vi "Embedded Project v3.vi"() -> ()   [LabVIEW 2015]
uses:
  <vilib>/Instr/_visa.llb/Select Event Type.ctl
  <vilib>/Instr/_visa.llb/VISA Configure Serial Port (Instr).vi
panel:
  in  "Tab Control":enum32{"Main", "Settings"}(tab)
  out "Node 3 Status":bool
  out "Node 2 Status":bool
  out "Bridge Stress":dbl[][](graph)
  out "Node 1 Status":bool
  out "Z Axis":dbl[][](graph)
  out "Y Axis":dbl[][](graph)
  out "X Axis":dbl[][](graph)
  out "Node 1 Water Level":u8(knob) scale=0.0..3.0
  out "Node 2 Water Level":u8(knob) scale=0.0..3.0
  out "Node 3 Water Level":u8(knob) scale=0.0..3.0
  out "Earthquake\nWarning":bool
  out "Tsunami \nWarning":bool
  out "Structure\nWarning":bool
  out "Serial Monitor":string
  out "System Time":string
  in  "COM Port":refnum<visa-resource-name>="COM1"
  in  "Terminate":bool
  out "Data Sorting":T1(array[cluster])
  out "New Serial Data":string
  # "Water Level Monitoring"
  # "Sensor Node Status"
  # "Earthquake Monitoring"
  # "Bridge Health Monitoring"
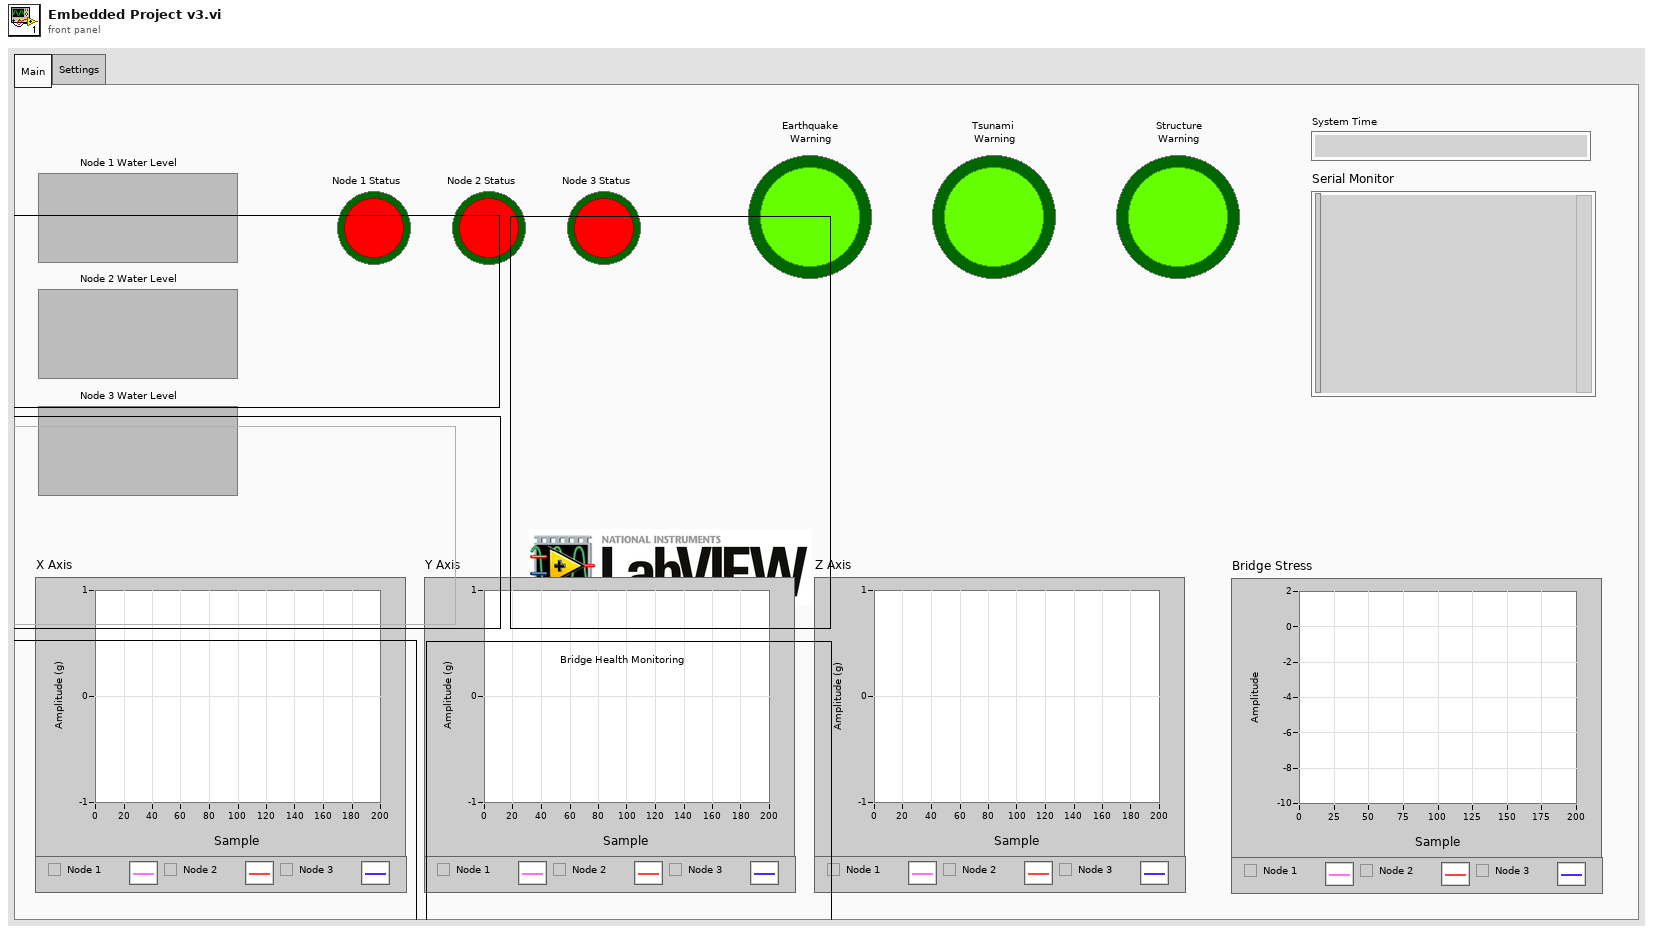
[diagram p1: front panel]
types:
  T1 = cluster{"Node Address":u16, "Water Level":i16, "Load Cell":i16, "Z Axis":i16, "Y Axis":i16, "X Axis":i16, "Status":u8}[]
  T2 = cluster{"Node Address":u16, "Water Level":i16, "Load Cell":i16, "X Axis":i16, "Y Axis":i16, "Z Axis":i16, "Status":u8}[]
  T3 = typedef "Select Event Type.ctl" = u32
  T4 = cluster{"baud rate (9600)":u32, "data bits (8)":u16, "parity (0:none)":enum16{"None", "Odd", "Even", "Mark", "Space"}, "stop bits (10: 1 bit)":u16, "flow control (0:none)":u16}
  T5 = cluster{"Node Address":u16, "Water Level":i16, "Load Cell":i16, "X Axis":i16, "Y Axis":i16, "Z Axis":i16, "Status":u8}
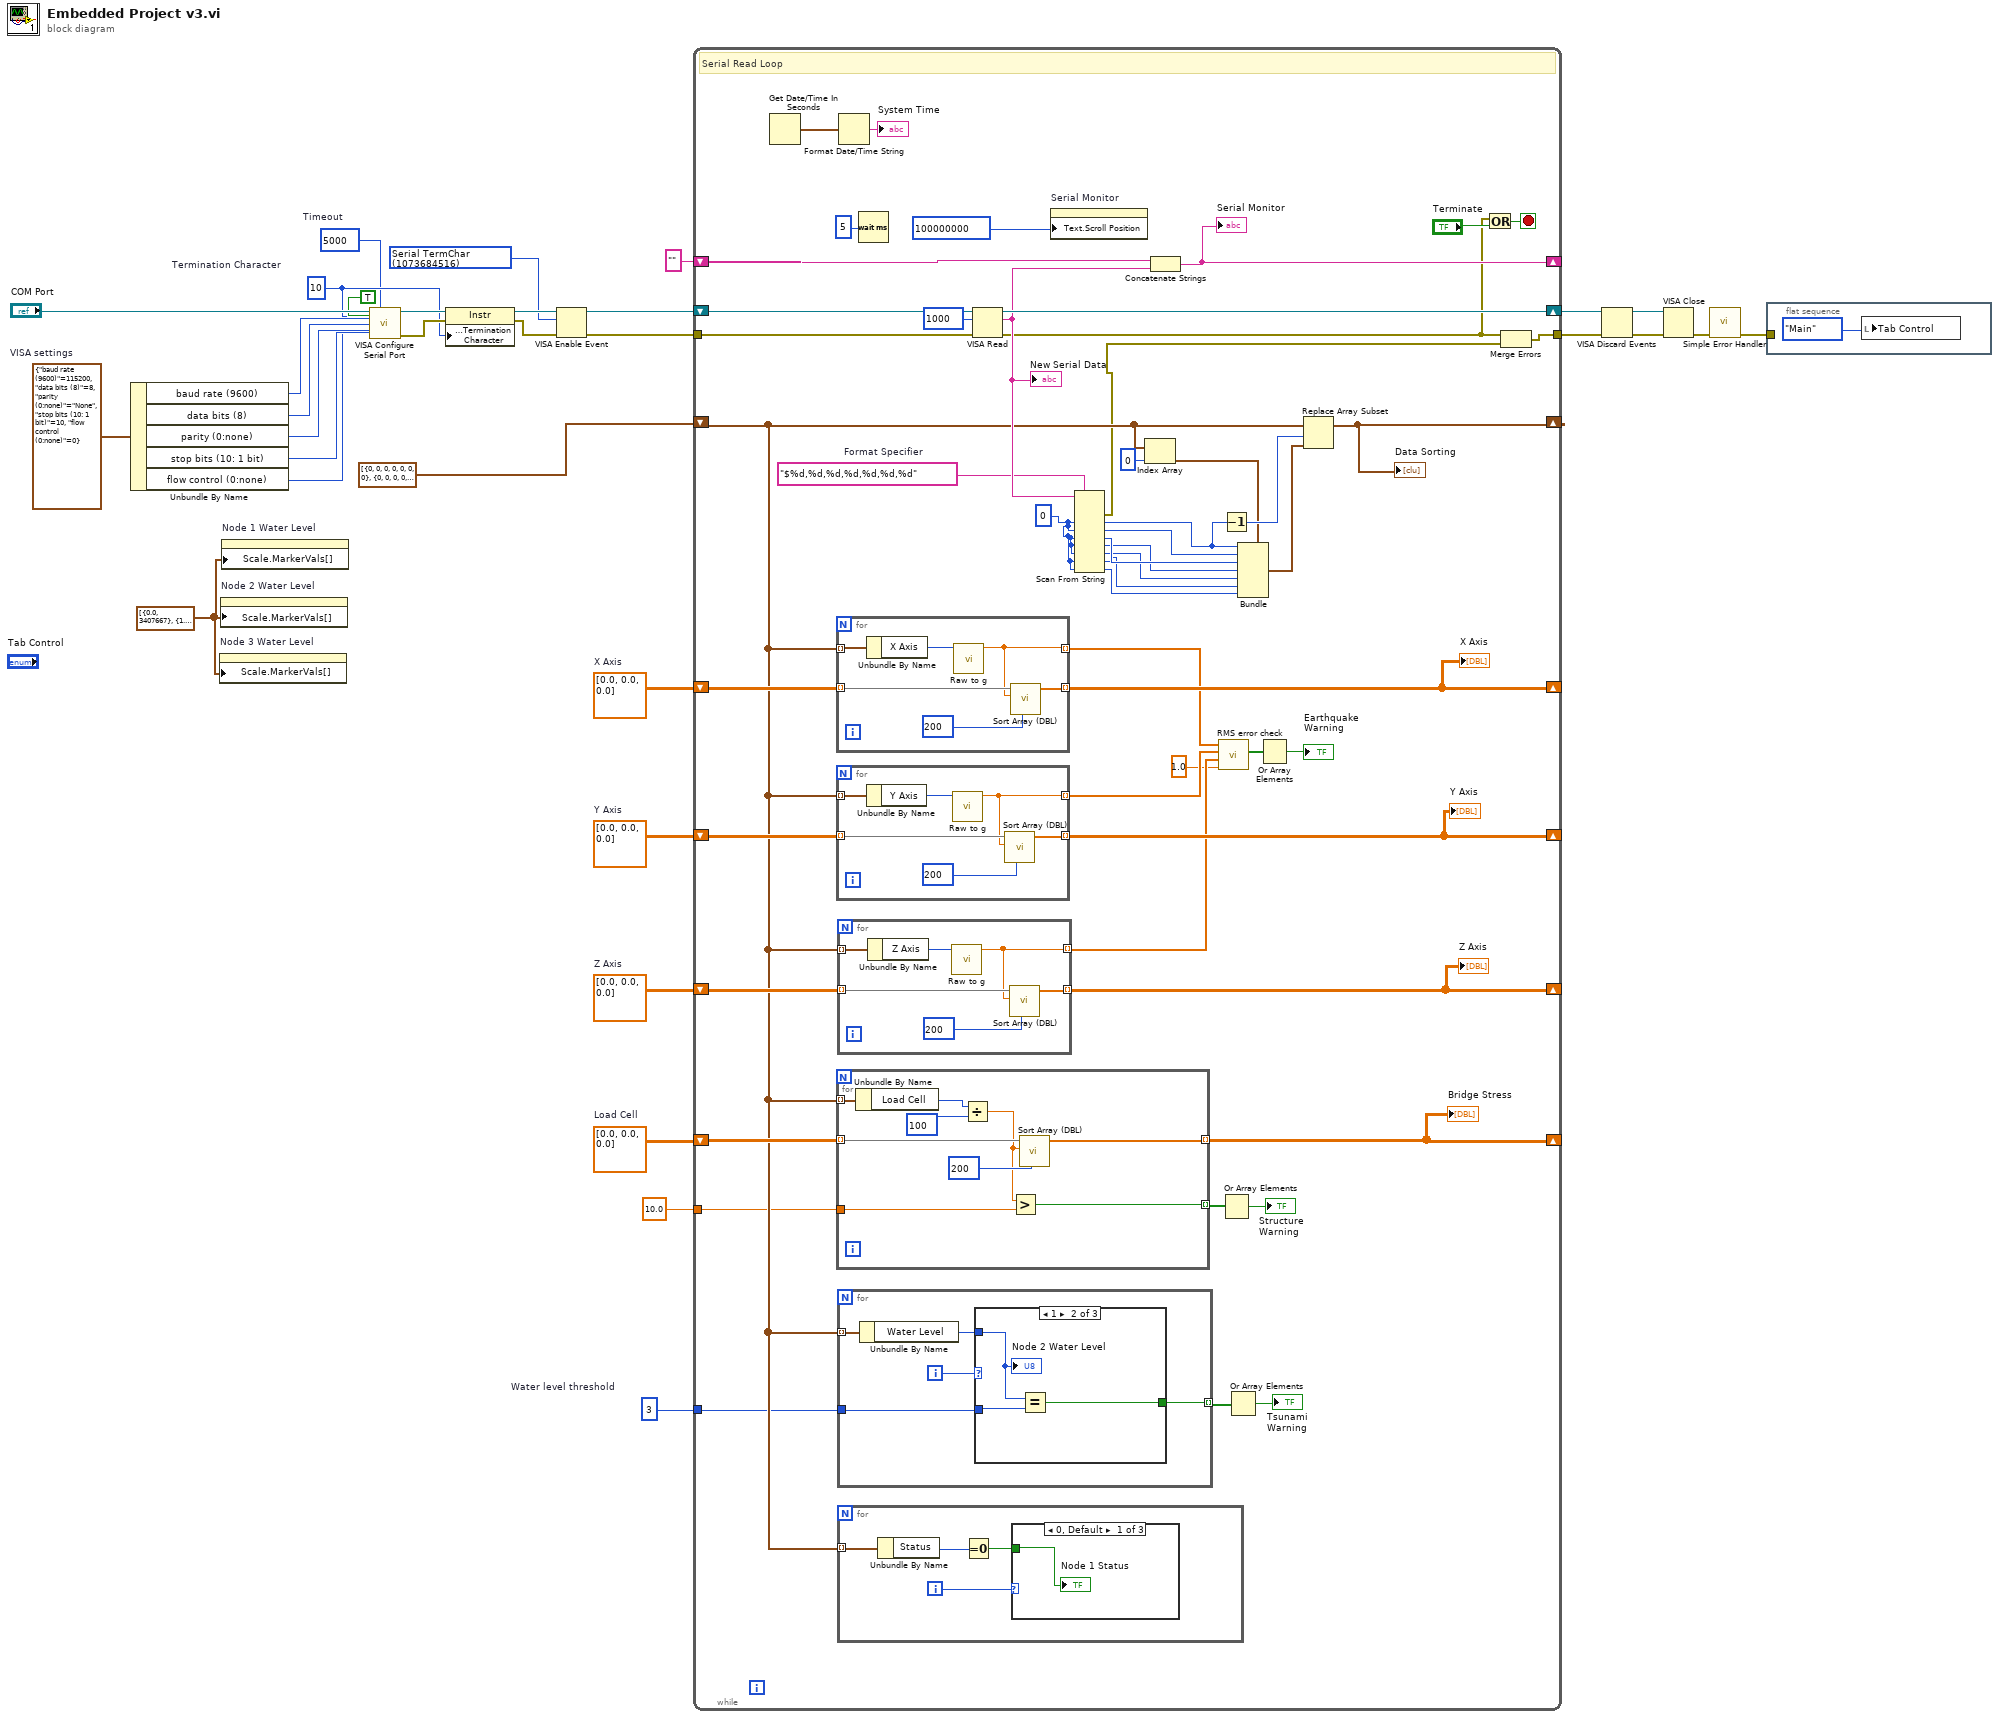
[diagram p0: block diagram]
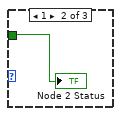
[diagram p2: hidden frame]
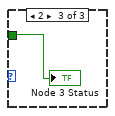
[diagram p3: hidden frame]
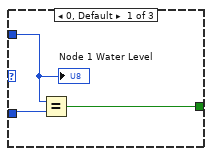
[diagram p4: hidden frame]
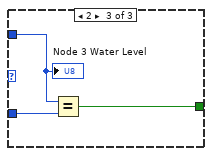
[diagram p5: hidden frame]
diagram:
  w2 = i16 3  # Water level threshold
  w3 = u32 5000  # Timeout
  w7 = cluster{dbl, u32}[] [{0.0, 3407667}, {1.0, 16777011}, {2.0, 16750899}, {3.0, 13369344}] ("Scale.Marker Values[]")
  w8 = dbl[][] [[0.0], [0.0], [0.0]]  # Load Cell
  w10 = dbl[][] [[0.0], [0.0], [0.0]]  # Z Axis
  w11 = dbl[][] [[0.0], [0.0], [0.0]]  # Y Axis
  w12 = dbl[][] [[0.0], [0.0], [0.0]]  # X Axis
  w18 = T3 1073684516 items=["Service Request"=1073684491, "Trigger"=3221168138, "Clear"=1073684493, "VXI Signal"=1073684512, "VXI/VME Interrupt"=3221168161, "VXI/VME Sysfail"=1073684509, "VXI/VME Sysreset"=1073684510, "GPIB CIC"=1073684498, "GPIB Talk"=1073684499, "GPIB Listen"=1073684500, "PXI Interrupt"=1073684514, "Serial Break"=1073684515, "Serial TermChar"=1073684516, "Serial CTS"=1073684521, "Serial DSR"=1073684522, "Serial DCD"=1073684524, "Serial RI"=1073684526, "Serial Character"=1073684533, "USB Interrupt"=1073684535, "All Enabled"=1073709055] ("Event Type")
  w28 = T4 {"baud rate (9600)"=115200, "data bits (8)"=8, "parity (0:none)"=enum."None", "stop bits (10: 1 bit)"=10, "flow control (0:none)"=0}  # VISA settings
  w21 = u8 10  # Termination Character
  n1 = Unbundle By Name(w28) -> ("baud rate (9600)"=w27:u32, "data bits (8)"=w26:u16, "parity (0:none)"=w25:enum16{"None", "Odd", "Even", "Mark", "Space"}, "stop bits (10: 1 bit)"=w24:u16, "flow control (0:none)"=w23:u16)
  n2 = property on="Node 3 Water Level" class="Knob (strict)"("Scale.MarkerVals[]"=w7) -> ()  [unwired: 2 in, 2 out]
  n3 = property on="Node 2 Water Level" class="Knob (strict)"("Scale.MarkerVals[]"=w7) -> ()  [unwired: 2 in, 2 out]
  n4 = property on="Node 1 Water Level" class="Knob (strict)"("Scale.MarkerVals[]"=w7) -> ()  [unwired: 2 in, 2 out]
  n5 = call-poly "VISA Configure Serial Port"("VISA resource name"="COM Port", "timeout (10sec)"=w3, "termination char\n(0xA = '\\n' = LF)"=w21, "Enable Termination\nChar (T)"=TRUE ("End Read on Termination Character?"), "baud rate (9600)"=w27, "data bits (8)"=w26, "parity (0:none)"=w25, "stop bits (10: 1 bit)"=w24, "flow control (0:none)"=w23) -> ("VISA resource name out"=w31:refnum<visa-resource-name>, "error out"=w22:errorcluster)  [unwired: 1 in, 4 out]
  n6 = property class="Instr"(reference=w31, error in=w22, "Message Based Settings:Termination Character"=w21) -> (reference out=w19:refnum<visa-resource-name>, error out=w20:errorcluster)
  n7 = VISA Enable Event(8:w20, 10:w18, 11:w19) -> (0:w5:errorcluster, 3:w6:refnum<visa-resource-name>)  [unwired: 1 in]
  n8 = while {
    shift-right: [w83] -> w16
    shift-left: w6 -> [w65]
    tunnel: [w50] -> w13
    shift-right: [w78] -> _
    shift-left: "" -> [w79]
    shift-right: [w76] -> _
    shift-left: T2 [{"Node Address"=0, "Water Level"=0, "Load Cell"=0, "X Axis"=0, "Y Axis"=0, "Z Axis"=0, "Status"=0}, {"Node Address"=0, "Water Level"=0, "Load Cell"=0, "X Axis"=0, "Y Axis"=0, "Z Axis"=0, "Status"=0}, {"Node Address"=0, "Water Level"=0, "Load Cell"=0, "X Axis"=0, "Y Axis"=0, "Z Axis"=0, "Status"=0}] ("Array") -> [w53]
    shift-right: [w46] -> _
    shift-left: w12 -> [w75]
    shift-right: [w47] -> _
    shift-left: w11 -> [w74]
    shift-right: [w45] -> _
    shift-left: w10 -> [w73]
    shift-right: [w70] -> _
    shift-left: w8 -> [w71]
    tunnel: w5 -> [w64]
    tunnel: w2 -> [w44]
    tunnel: 10.0 ("y") -> [w41]
    stop <- w81 stop-if-true
    w60 = i16 0 ("default value 1")
    w67 = "$%d,%d,%d,%d,%d,%d,%d"  # Format Specifier
    # "Serial Read Loop"
    n9 = Get Date/Time In Seconds() -> (seconds since 1Jan1904=w69:timestamp)
    n10 = for {
      tunnel: w53 -> [w131] mode=indexing
      tunnel: w75 -> [w129] mode=indexing
      tunnel: [w128] -> w46 mode=indexing
      tunnel: [w126] -> w38 mode=indexing
      n11 = Unbundle By Name(w131) -> ("X Axis"=w130:i16)
      n12 = call "Raw to g.vi"("Input"=w130) -> ("Output"=w126:dbl)  [unwired: 10 in]
      n13 = call "Sort Array (DBL).vi"("Max Size"=200, "New Element"=w126, "Array In"=w129) -> ("Array Out"=w128:dbl[])  [unwired: 8 in]
    }
    "X Axis" <- w46
    n14 = for {
      tunnel: w74 -> [w123] mode=indexing
      tunnel: w53 -> [w125] mode=indexing
      tunnel: [w122] -> w47 mode=indexing
      tunnel: [w120] -> w37 mode=indexing
      n15 = Unbundle By Name(w125) -> ("Y Axis"=w124:i16)
      n16 = call "Raw to g.vi"("Input"=w124) -> ("Output"=w120:dbl)  [unwired: 10 in]
      n17 = call "Sort Array (DBL).vi"("Max Size"=200, "New Element"=w120, "Array In"=w123) -> ("Array Out"=w122:dbl[])  [unwired: 8 in]
    }
    "Y Axis" <- w47
    n18 = for {
      tunnel: [w112] -> w70 mode=indexing
      tunnel: w71 -> [w111] mode=indexing
      tunnel: w53 -> [w113] mode=indexing
      tunnel: w41 -> [w106]
      tunnel: [w105] -> w40 mode=indexing
      n19 = Unbundle By Name(w113) -> ("Load Cell"=w109:i16)
      n20 = Divide(x=w109, y=i16 100) -> (x/y=w107:dbl)
      n21 = Greater?(x=w107, y=w106) -> (0:w105:bool)
      n22 = call "Sort Array (DBL).vi"("Max Size"=200, "New Element"=w107, "Array In"=w111) -> ("Array Out"=w112:dbl[])  [unwired: 8 in]
    }
    "Bridge Stress" <- w70
    n23 = for {
      tunnel: w73 -> [w117] mode=indexing
      tunnel: w53 -> [w119] mode=indexing
      tunnel: [w116] -> w45 mode=indexing
      tunnel: [w114] -> w36 mode=indexing
      n24 = Unbundle By Name(w119) -> ("Z Axis"=w118:i16)
      n25 = call "Raw to g.vi"("Input"=w118) -> ("Output"=w114:dbl)  [unwired: 10 in]
      n26 = call "Sort Array (DBL).vi"("Max Size"=200, "New Element"=w114, "Array In"=w117) -> ("Array Out"=w116:dbl[])  [unwired: 8 in]
    }
    "Z Axis" <- w45
    n27 = for {
      tunnel: w53 -> [w95] mode=indexing
      tunnel: w44 -> [w92]
      tunnel: [w91] -> w43 mode=indexing
      i -> [w94]
      n28 = Unbundle By Name(w95) -> ("Water Level"=w93:i16)
      n29 = case shown="1" w94 {
        tunnel: w93 -> [w98 w101 w104]
        tunnel: w92 -> [w96 w99 w103]
        tunnel: [w97 w100 w102] -> w91
        frame 0, Default {
          n30 = Equal?(x=w98, y=w96) -> (x = y?=w97:bool)
          "Node 1 Water Level" <- w98
        }
        frame 1 {
          n31 = Equal?(x=w101, y=w99) -> (x = y?=w100:bool)
          "Node 2 Water Level" <- w101
        }
        frame 2 {
          n32 = Equal?(x=w104, y=w103) -> (x = y?=w102:bool)
          "Node 3 Water Level" <- w104
        }
      }
    }
    n33 = for {
      tunnel: w53 -> [w87] mode=indexing
      i -> [w86]
      n34 = Unbundle By Name(w87) -> ("Status"=w85:u8)
      n35 = Equal To 0?(x=w85) -> (x = 0?=w84:bool)
      n36 = case shown="0, Default" w86 {
        tunnel: w84 -> [w88 w89 w90]
        frame 0, Default {
          "Node 1 Status" <- w88
        }
        frame 1 {
          "Node 2 Status" <- w89
        }
        frame 2 {
          "Node 3 Status" <- w90
        }
      }
    }
    n37 = Format Date/Time String(seconds (now)=w69) -> (date/time string=→"System Time":string)  [unwired: 2 in]
    n38 = Wait (ms)(milliseconds to wait=u32 5) -> ()  [unwired: 1 out]
    n39 = VISA Read(VISA resource name=w65, byte count=u32 1000, error in (no error)=w64) -> (VISA resource name out=w83:refnum<visa-resource-name>, read buffer=w77:string, error out=w49:errorcluster)  [unwired: 1 out]
    "New Serial Data" <- w77
    n40 = property on="Serial Monitor" class="Str"("Text.Scroll Position"=u32 100000000) -> ()  [unwired: 2 in, 2 out]
    n41 = Scan From String(format string=w67, input string=w77, default 1=w60, default 2=w60, default 3=w60, default 4=w60, default 5=w60, default 6=w60, default 7=w60) -> (error out=w48:errorcluster, output 1=w66:i16, output 2=w59:i16, output 3=w58:i16, output 4=w57:i16, output 5=w56:i16, output 6=w55:i16, output 7=w54:i16)  [unwired: 2 in, 2 out]
    n42 = Index Array(array=w53, index=0) -> (element=w51:T5)
    n43 = Concatenate Strings(w79, w77) -> (w78:string)
    "Serial Monitor" <- w78
    n44 = call "RMS error check.vi"("Threshold"=1.0, "Z Axis"=w36, "Y Axis"=w37, "X Axis"=w38) -> ("Error?"=w34:bool[])  [unwired: 6 in, 1 out]
    n45 = Decrement(x=w66) -> (x-1=w62:i16)
    n46 = Or Array Elements(Boolean array=w40) -> (logical OR=→"Structure\nWarning":bool)
    n47 = Or Array Elements(Boolean array=w43) -> (logical OR=→"Tsunami \nWarning":bool)
    n48 = Bundle(cluster=w51, "Node Address"=w66, "Water Level"=w59, "Load Cell"=w58, "X Axis"=w57, "Y Axis"=w56, "Z Axis"=w55, "Status"=w54) -> (w61:T5)
    n49 = Or Array Elements(Boolean array=w34) -> (logical OR=→"Earthquake\nWarning":bool)
    n50 = Replace Array Subset(array=w53, new element=w61, index=w62) -> (w76:T2)
    "Data Sorting" <- w76
    n51 = Or(x=w49, y="Terminate") -> (x .or. y?=w81:bool)
    n52 = Merge Errors(w49, w48) -> (w50:errorcluster)
  }
  n53 = VISA Discard Events(8:w13, 11:w16) -> (0:w14:errorcluster, 3:w15:refnum<visa-resource-name>)  [unwired: 2 in]
  n54 = VISA Close(VISA resource name=w15, error in (no error)=w14) -> (error out=w29:errorcluster)
  n55 = call <vilib>:"Simple Error Handler.vi"("error in (no error)"=w29) -> ("error out"=w4:errorcluster)  [unwired: 1 in, 7 out]
  n56 = flat-sequence {
    tunnel: w4 -> [_]
    frame #0 {
      n57 = local write "Tab Control"(enum32{"Main", "Settings"}."Main" ("Tab Control")) -> ()
    }
  }
